vi "ParseMsg.vi"(2 "Buf Len":u16, 3 "Input Buffer":u8[](array[numeric])) -> ()   [LabVIEW 2016]
uses:
  RcvMsgType.ctl
  GlobalVars.vi
panel:
  in  "Rcv Msg Type":T1={"ID"=135, "Chksum"=123, "Unused"=0, "Length"=0, "Seq No"=0, "Msg Data"=[]}
  in  "Buf Idx":u16
  out "Temp":u8
  in  "Done":bool
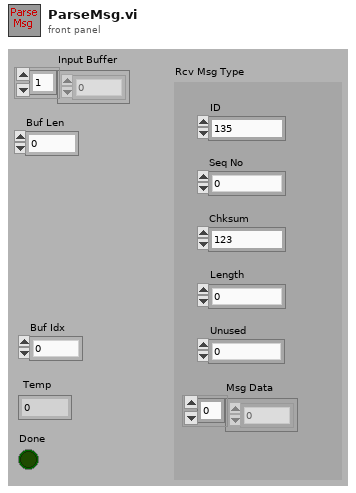
[diagram p1: front panel]
types:
  T1 = typedef "RcvMsgType.ctl" = cluster{"ID":u8, "Chksum":u16, "Unused":u16, "Length":u16, "Seq No":u8, "Msg Data":u8[]}
  T2 = typedef "Queue RefNum" = refnum<k1>
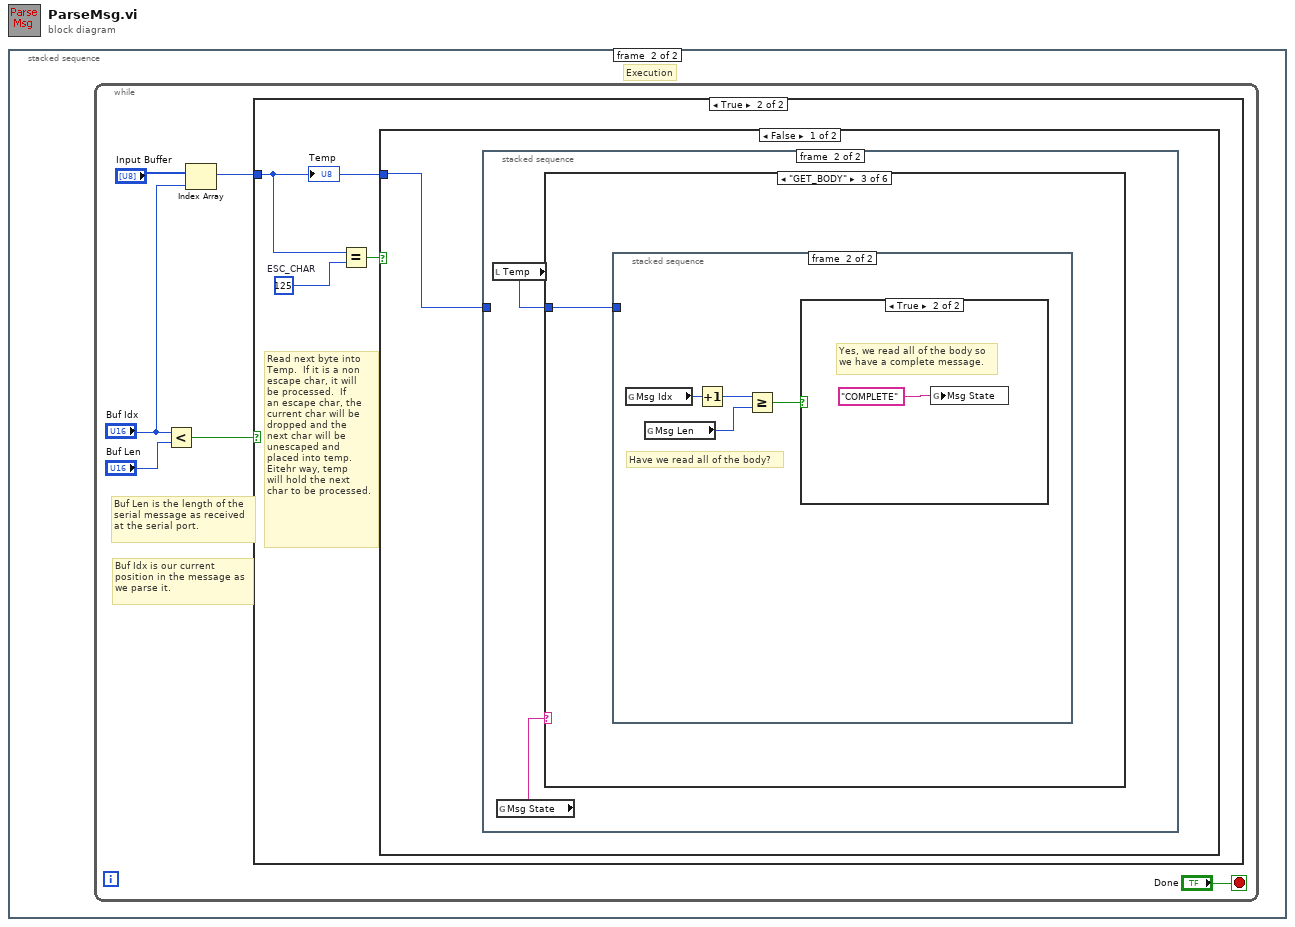
[diagram p0: block diagram]
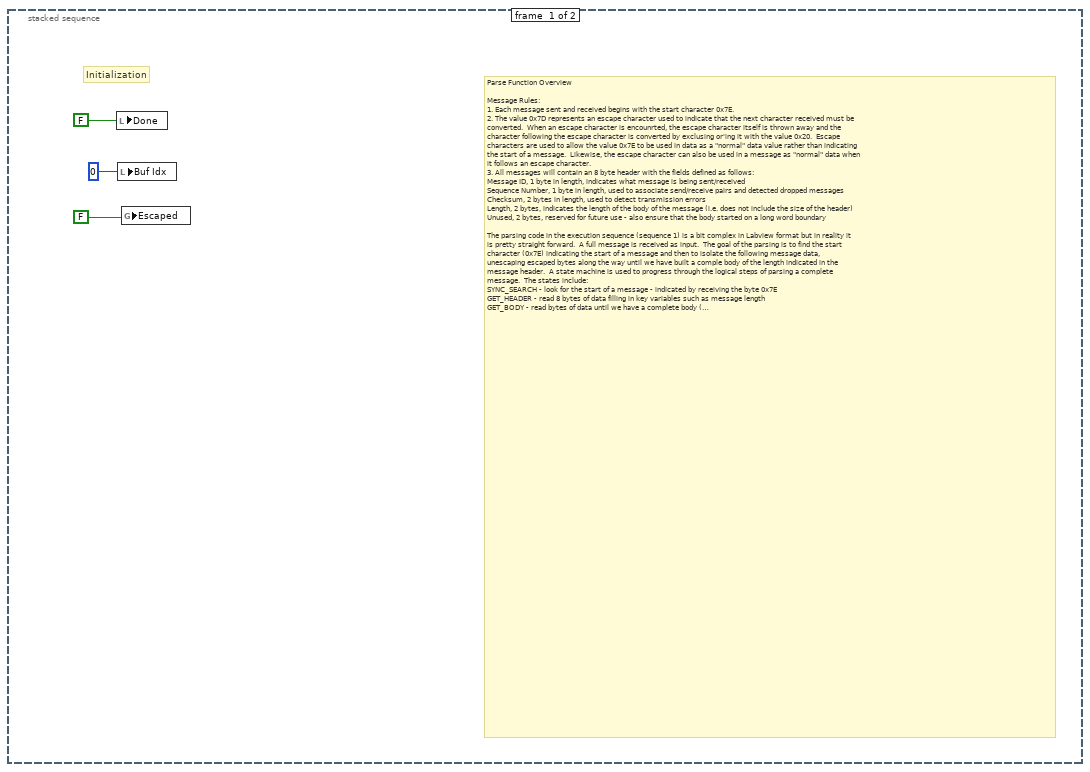
[diagram p2: hidden frame]
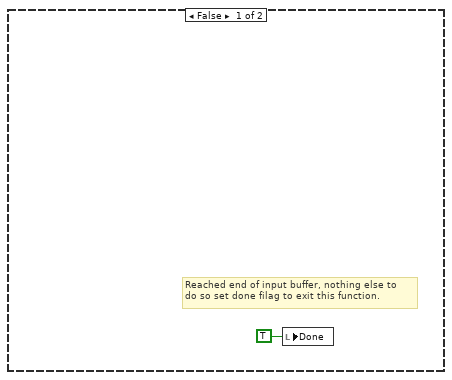
[diagram p3: hidden frame]
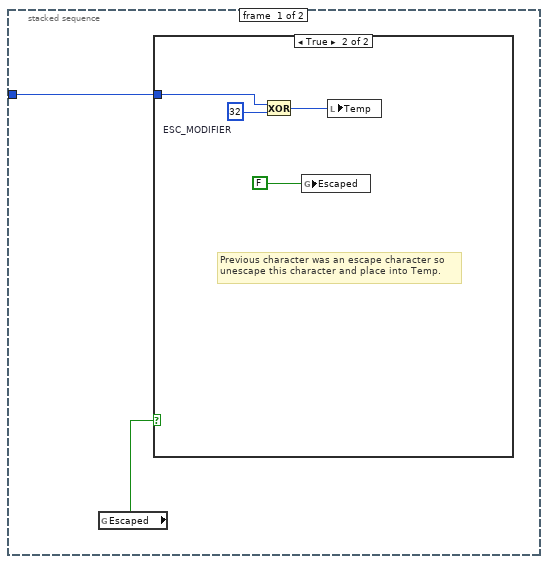
[diagram p4: hidden frame]
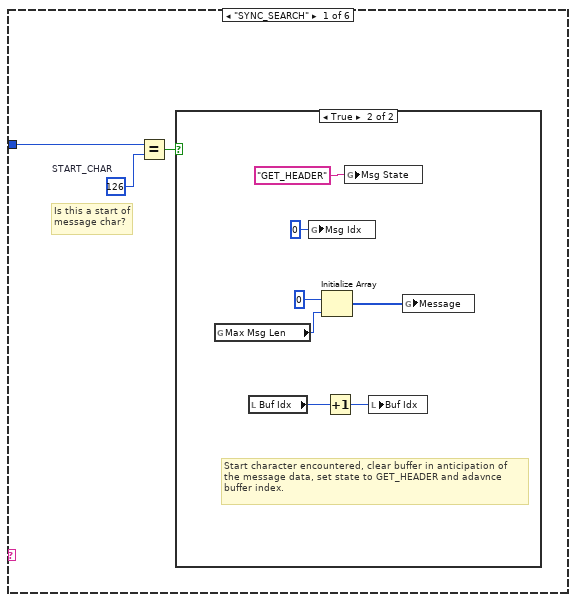
[diagram p6: hidden frame]
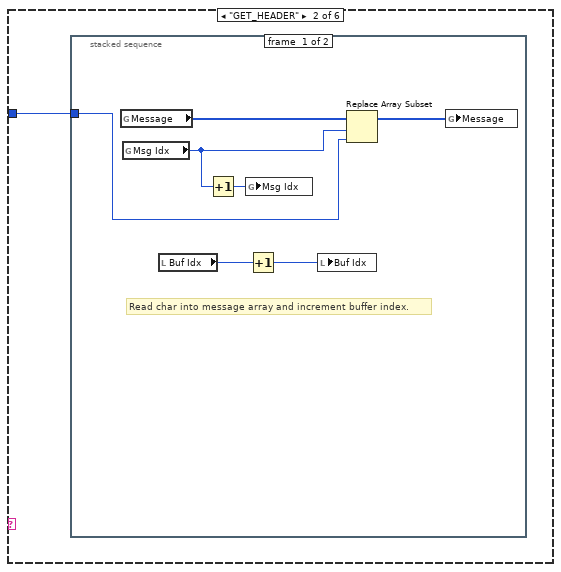
[diagram p8: hidden frame]
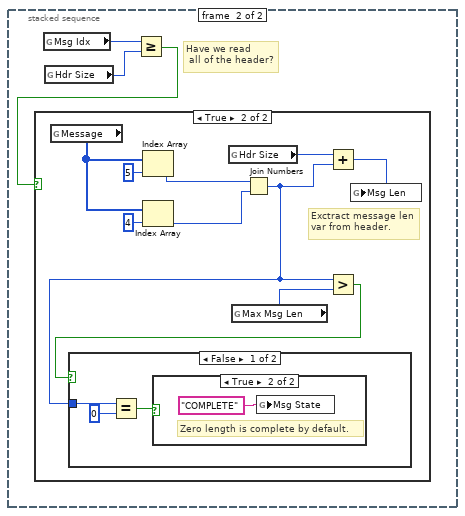
[diagram p9: hidden frame]
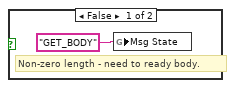
[diagram p11: hidden frame]
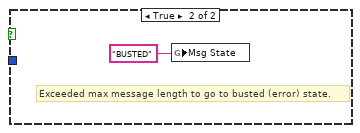
[diagram p12: hidden frame]
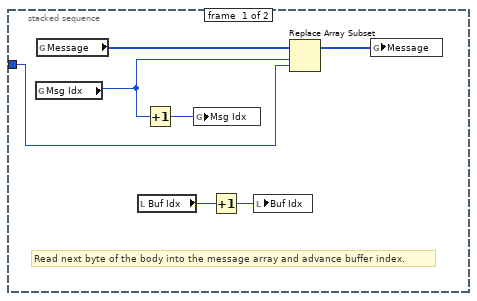
[diagram p13: hidden frame]
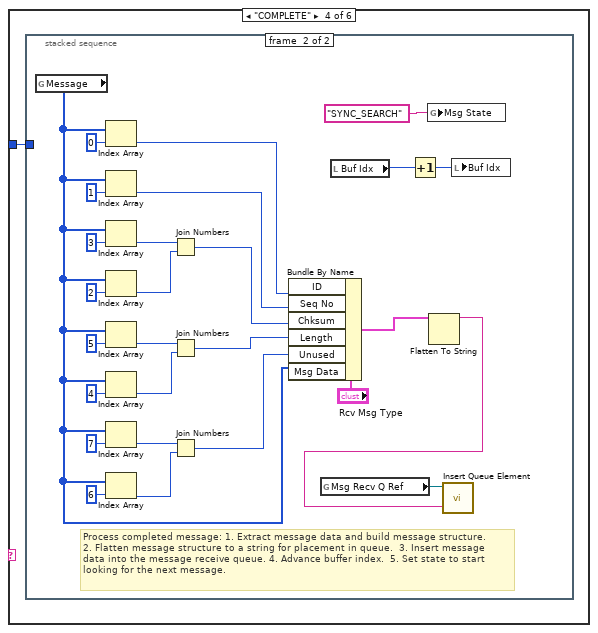
[diagram p15: hidden frame]
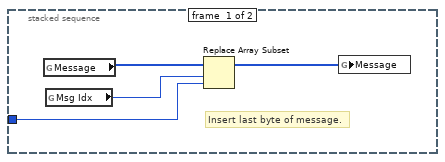
[diagram p16: hidden frame]
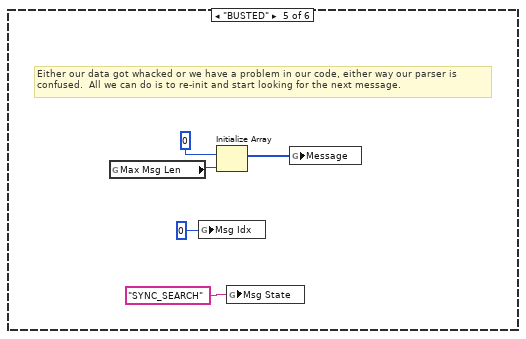
[diagram p17: hidden frame]
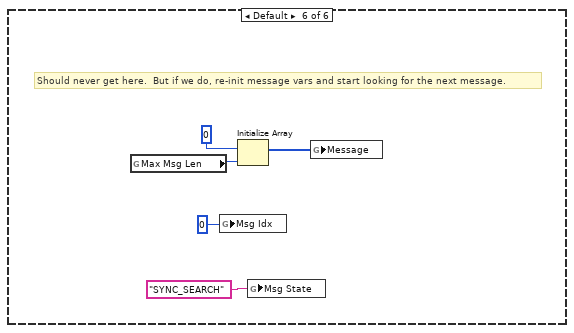
[diagram p18: hidden frame]
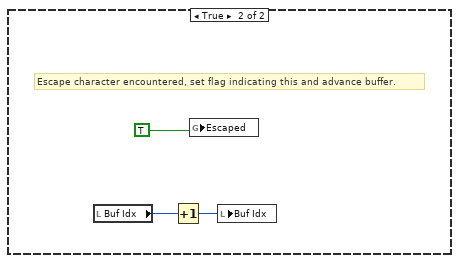
[diagram p19: hidden frame]
diagram:
  n1 = stacked-sequence {
    frame #0 {
      # "Parse Function Overview\n\nMessage Rules:\n1. Each message sent and received begins with the start character 0x7E.\n2. The value 0x7D represents an escape character used to indicate that the next character received must be\nconverted.  When an escape character is encounrted, the escape character itself is thrown away and the\ncharacter following the escape character is converted by exclusing or'ing it with the value 0x20.  Escape\ncharacters are used to allow the value 0x7E to be used in data as a \"normal\" data value rather than indicating\nthe start of a message.  Likewise, the escape character can also be used in a message as \"normal\" data when\nit follows an escape character.\n3. All messages will contain an 8 byte header with the fields defined as follows:\nMessage ID, 1 byte in length, indicates what message is being sent/received\nSequence Number, 1 byte in length, used to associate send/receive pairs and detected dropped messages\nChecksum, 2 bytes in length, used to detect transmission errors\nLength, 2 bytes, indicates the length of the body of the message (i.e. does not include the size of the header)\nUnused, 2 bytes, reserved for future use - also ensure that the body started on a long word boundary\n\nThe parsing code in the execution sequence (sequence 1) is a bit complex in Labview format but in reality it\nis pretty straight forward.  A full message is received as input.  The goal of the parsing is to find the start\ncharacter (0x7E) indicating the start of a message and then to isolate the following message data,\nunescaping escaped bytes along the way until we have built a comple body of the length indicated in the\nmessage header.  A state machine is used to progress through the logical steps of parsing a complete\nmessage.  The states include:\nSYNC_SEARCH - look for the start of a message - indicated by receiving the byte 0x7E\nGET_HEADER - read 8 bytes of data filling in key variables such as message length\nGET_BODY - read bytes of data until we have a complete body (i.e. message length bytes)\nCOMPLETE - we have a full message - transfer data to message structure and put on receive queue\nBUSTED - if we encounter an error go to this state - it reinitializes for pasing the next message\nDefault - should never happen but if it does reinitialized for parsing the next message\n\nEach state progress to the next state once it find what it is looking for.  State transitions are as follows:\nSYNC_SEARCH -> GET_HEADER\nGET_HEADER -> GET_BODY, BUSTED on error\nGET_BODY -> COMPLETE, BUSTED on error\nCOMPLETE -> SYNC_SEARCH\n\nFor each byte received, if it is an escape character, set a flag indicating this so the next character received\ncan be unescpaed.  The escpae character itself is discarded.\n\nIt is important to know that this function supports receiving a single complete message as well as both\npartial and multiple messages as there is no guarantee that the received serial packets will contain\nexactly one complete message.  As such, global variables had to be utilzed to maintain parsing state\nfrom one invocation to the next."
      # "Initialization"
      n2 = local write "Done"(FALSE ("Done")) -> ()
      n3 = local write "Buf Idx"(u32 0 ("Buf Pos")) -> ()
      n4 = global write "GlobalVars.vi" "Escaped"(FALSE ("Escaped")) -> ()
    }
    frame #1 {
      # "Execution"
      n5 = while {
        stop <- "Done" stop-if-true
        # "Buf Idx is our current\nposition in the message as\nwe parse it."
        # "Buf Len is the length of the\nserial message as received\nat the serial port."
        n6 = Less?(x="Buf Idx", y="Buf Len") -> (x < y?=w8:bool)
        n7 = Index Array "Index Array"(array="Input Buffer", index="Buf Idx") -> (element=w5:u8)
        n8 = case shown="True" w8 {
          tunnel: w5 -> [_ w11]
          frame False {
            # "Reached end of input buffer, nothing else to\ndo so set done filag to exit this function."
            n9 = local write "Done"(TRUE ("Done")) -> ()
          }
          frame True {
            w13 = u8 125  # ESC_CHAR
            # "Read next byte into\nTemp.  If it is a non\nescape char, it will\nbe processed.  If\nan escape char, the\ncurrent char will be\ndropped and the\nnext char will be \nunescaped and\nplaced into temp.\nEitehr way, temp\nwill hold the next\nchar to be processed."
            n10 = Equal?(x=w11, y=w13) -> (x = y?=w12:bool)
            n11 = case shown="False" w12 {
              tunnel: w11 -> [w14 _]
              frame False {
                n12 = stacked-sequence {
                  tunnel: w14 -> [w16 _]
                  frame #0 {
                    n13 = global read "GlobalVars.vi" "Escaped"() -> (w15:bool)
                    n14 = case shown="True" w15 {
                      tunnel: w16 -> [_ w19]
                      frame False {
                      }
                      frame True {
                        w20 = u8 32  # ESC_MODIFIER
                        # "Previous character was an escape character so\nunescape this character and place into Temp."
                        n15 = Exclusive Or(1:w20, 2:w19) -> (0:w18:u8)
                        n16 = global write "GlobalVars.vi" "Escaped"(FALSE ("Escaped")) -> ()
                        n17 = local write "Temp"(w18) -> ()
                      }
                    }
                  }
                  frame #1 {
                    n18 = local read "Temp"() -> (w21:u8)
                    n19 = global read "GlobalVars.vi" "Msg State"() -> (w22:string)
                    n20 = case shown="\"GET_BODY\"" w22 {
                      tunnel: w21 -> [w25 w33 w60 w73 _ _]
                      frame "SYNC_SEARCH" {
                        w24 = u8 126  # START_CHAR
                        # "Is this a start of\nmessage char?"
                        n21 = Equal?(x=w25, y=w24) -> (x = y?=w23:bool)
                        n22 = case shown="True" w23 {
                          frame False {
                          }
                          frame True {
                            # "Start character encountered, clear buffer in anticipation of\nthe message data, set state to GET_HEADER and adavnce\nbuffer index."
                            n23 = global read "GlobalVars.vi" "Max Msg Len"() -> (w30:u16)
                            n24 = local read "Buf Idx"() -> (w27:u16)
                            n25 = global write "GlobalVars.vi" "Msg Idx"(u32 0 ("Msg_Pos")) -> ()
                            n26 = Initialize Array "Initialize Array"(u8 0 ("Element Data"), w30) -> (w28:u8[])
                            n27 = Increment(x=w27) -> (x+1=w26:u16)
                            n28 = global write "GlobalVars.vi" "Msg State"("GET_HEADER" ("Msg State")) -> ()
                            n29 = local write "Buf Idx"(w26) -> ()
                            n30 = global write "GlobalVars.vi" "Message"(w28) -> ()
                          }
                        }
                      }
                      frame "GET_HEADER" {
                        n31 = stacked-sequence {
                          tunnel: w33 -> [w37 _]
                          frame #0 {
                            # "Read char into message array and increment buffer index."
                            n32 = global read "GlobalVars.vi" "Message"() -> (w40:u8[])
                            n33 = global read "GlobalVars.vi" "Msg Idx"() -> (w36:u32)
                            n34 = local read "Buf Idx"() -> (w35:u16)
                            n35 = Increment(x=w36) -> (x+1=w38:u32)
                            n36 = global write "GlobalVars.vi" "Msg Idx"(w38) -> ()
                            n37 = Increment(x=w35) -> (x+1=w34:u16)
                            n38 = local write "Buf Idx"(w34) -> ()
                            n39 = Replace Array Subset "Replace Array Subset"(array=w40, new element=w37, index=w36) -> (w39:u8[])
                            n40 = global write "GlobalVars.vi" "Message"(w39) -> ()
                          }
                          frame #1 {
                            # "Have we read\n all of the header?"
                            n41 = global read "GlobalVars.vi" "Msg Idx"() -> (w43:u32)
                            n42 = global read "GlobalVars.vi" "Hdr Size"() -> (w41:u8)
                            n43 = Greater Or Equal?(x=w43, y=w41) -> (x >= y?=w42:bool)
                            n44 = case shown="True" w42 {
                              frame False {
                              }
                              frame True {
                                # "Exctract message len\nvar from header."
                                n45 = global read "GlobalVars.vi" "Message"() -> (w53:u8[])
                                n46 = Index Array "Index Array"(array=w53, index=5 ("Index")) -> (element=w50:u8)
                                n47 = Index Array "Index Array"(array=w53, index=4 ("Index")) -> (element=w49:u8)
                                n48 = global read "GlobalVars.vi" "Hdr Size"() -> (w45:u8)
                                n49 = global read "GlobalVars.vi" "Max Msg Len"() -> (w48:u16)
                                n50 = Join Numbers(hi=w50, lo=w49) -> ((hi.lo)=w44:u16)
                                n51 = Add(x=w45, y=w44) -> (x+y=w46:u16)
                                n52 = Greater?(x=w44, y=w48) -> (0:w47:bool)
                                n53 = case shown="False" w47 {
                                tunnel: w44 -> [w56 _]
                                frame False {
                                n54 = Equal?(x=w56, y=u16 0) -> (x = y?=w54:bool)
                                n55 = case shown="True" w54 {
                                frame False {
                                # "Non-zero length - need to ready body."
                                n56 = global write "GlobalVars.vi" "Msg State"("GET_BODY" ("Msg State")) -> ()
                                }
                                frame True {
                                # "Zero length is complete by default."
                                n57 = global write "GlobalVars.vi" "Msg State"("COMPLETE" ("Msg State")) -> ()
                                }
                                }
                                }
                                frame True {
                                # "Exceeded max message length to go to busted (error) state."
                                n58 = global write "GlobalVars.vi" "Msg State"("BUSTED" ("Msg State")) -> ()
                                }
                                }
                                n59 = global write "GlobalVars.vi" "Msg Len"(w46) -> ()
                              }
                            }
                          }
                        }
                      }
                      frame "GET_BODY" {
                        n60 = stacked-sequence {
                          tunnel: w60 -> [w61 _]
                          frame #0 {
                            # "Read next byte of the body into the message array and advance buffer index."
                            n61 = global read "GlobalVars.vi" "Msg Idx"() -> (w62:u32)
                            n62 = global read "GlobalVars.vi" "Message"() -> (w65:u8[])
                            n63 = local read "Buf Idx"() -> (w67:u16)
                            n64 = Increment(x=w62) -> (x+1=w63:u32)
                            n65 = global write "GlobalVars.vi" "Msg Idx"(w63) -> ()
                            n66 = Increment(x=w67) -> (x+1=w66:u16)
                            n67 = local write "Buf Idx"(w66) -> ()
                            n68 = Replace Array Subset "Replace Array Subset"(array=w65, new element=w61, index=w62) -> (w64:u8[])
                            n69 = global write "GlobalVars.vi" "Message"(w64) -> ()
                          }
                          frame #1 {
                            # "Have we read all of the body?"
                            n70 = global read "GlobalVars.vi" "Msg Idx"() -> (w69:u32)
                            n71 = global read "GlobalVars.vi" "Msg Len"() -> (w71:u32)
                            n72 = Increment(x=w69) -> (x+1=w68:u32)
                            n73 = Greater Or Equal?(x=w68, y=w71) -> (x >= y?=w70:bool)
                            n74 = case shown="True" w70 {
                              frame False {
                              }
                              frame True {
                                # "Yes, we read all of the body so\nwe have a complete message."
                                n75 = global write "GlobalVars.vi" "Msg State"("COMPLETE" ("Msg State")) -> ()
                              }
                            }
                          }
                        }
                      }
                      frame "COMPLETE" {
                        n76 = stacked-sequence {
                          tunnel: w73 -> [w75 _]
                          frame #0 {
                            # "Insert last byte of message."
                            n77 = global read "GlobalVars.vi" "Message"() -> (w77:u8[])
                            n78 = global read "GlobalVars.vi" "Msg Idx"() -> (w76:u32)
                            n79 = Replace Array Subset "Replace Array Subset"(array=w77, new element=w75, index=w76) -> (w74:u8[])
                            n80 = global write "GlobalVars.vi" "Message"(w74) -> ()
                          }
                          frame #1 {
                            # "Process completed message: 1. Extract message data and build message structure.\n2. Flatten message structure to a string for placement in queue.  3. Insert message\ndata into the message receive queue. 4. Advance buffer index.  5. Set state to start\nlooking for the next message."
                            n81 = global read "GlobalVars.vi" "Message"() -> (w88:u8[])
                            n82 = Index Array "Index Array"(array=w88, index=0 ("Index")) -> (element=w83:u8)
                            n83 = Index Array "Index Array"(array=w88, index=1 ("Index")) -> (element=w84:u8)
                            n84 = Index Array "Index Array"(array=w88, index=3 ("Index")) -> (element=w96:u8)
                            n85 = Index Array "Index Array"(array=w88, index=2 ("Index")) -> (element=w95:u8)
                            n86 = Index Array "Index Array"(array=w88, index=5 ("Index")) -> (element=w94:u8)
                            n87 = Index Array "Index Array"(array=w88, index=4 ("Index")) -> (element=w93:u8)
                            n88 = Index Array "Index Array"(array=w88, index=7 ("Index")) -> (element=w92:u8)
                            n89 = Index Array "Index Array"(array=w88, index=6 ("Index")) -> (element=w91:u8)
                            n90 = Join Numbers(hi=w96, lo=w95) -> ((hi.lo)=w85:u16)
                            n91 = Join Numbers(hi=w94, lo=w93) -> ((hi.lo)=w86:u16)
                            n92 = Join Numbers(hi=w92, lo=w91) -> ((hi.lo)=w87:u16)
                            n93 = Bundle By Name(cluster="Rcv Msg Type", "ID"=w83, "Seq No"=w84, "Chksum"=w85, "Length"=w86, "Unused"=w87, "Msg Data"=w88) -> (w82:T1)
                            n94 = global read "GlobalVars.vi" "Msg Recv Q Ref"() -> (w90:T2)
                            n95 = local read "Buf Idx"() -> (w79:u16)
                            n96 = Increment(x=w79) -> (x+1=w78:u16)
                            n97 = global write "GlobalVars.vi" "Msg State"("SYNC_SEARCH" ("Msg State")) -> ()
                            n98 = Flatten To String(anything=w82) -> (data string=w89:string)  [unwired: 3 in, 2 out]
                            n99 = call <vilib>:"Insert Queue Element.vi"("queue element"=w89, "queue"=w90) -> ()  [unwired: 5 in, 3 out]
                            n100 = local write "Buf Idx"(w78) -> ()
                          }
                        }
                      }
                      frame "BUSTED" {
                        # "Either our data got whacked or we have a problem in our code, either way our parser is\nconfused.  All we can do is to re-init and start looking for the next message."
                        n101 = global read "GlobalVars.vi" "Max Msg Len"() -> (w108:u16)
                        n102 = global write "GlobalVars.vi" "Msg Idx"(u32 0 ("Msg Idx")) -> ()
                        n103 = Initialize Array "Initialize Array"(u8 0 ("Element Data"), w108) -> (w109:u8[])
                        n104 = global write "GlobalVars.vi" "Msg State"("SYNC_SEARCH" ("Msg State")) -> ()
                        n105 = global write "GlobalVars.vi" "Message"(w109) -> ()
                      }
                      frame Default {
                        # "Should never get here.  But if we do, re-init message vars and start looking for the next message."
                        n106 = global read "GlobalVars.vi" "Max Msg Len"() -> (w113:u16)
                        n107 = global write "GlobalVars.vi" "Msg Idx"(u32 0 ("Msg Idx")) -> ()
                        n108 = Initialize Array "Initialize Array"(u8 0 ("Element Data"), w113) -> (w114:u8[])
                        n109 = global write "GlobalVars.vi" "Msg State"("SYNC_SEARCH" ("Msg State")) -> ()
                        n110 = global write "GlobalVars.vi" "Message"(w114) -> ()
                      }
                    }
                  }
                }
              }
              frame True {
                # "Escape character encountered, set flag indicating this and advance buffer."
                n111 = local read "Buf Idx"() -> (w117:u16)
                n112 = Increment(x=w117) -> (x+1=w116:u16)
                n113 = global write "GlobalVars.vi" "Escaped"(TRUE ("Escaped")) -> ()
                n114 = local write "Buf Idx"(w116) -> ()
              }
            }
            "Temp" <- w11
          }
        }
      }
    }
  }
